vi "IsAnyOfType.vi"(8 "error in (no error)":errorcluster, 9 "Message Type":string, 10 "Any":T1, 11 "gRPCid in":T2) -> (0 "error out":errorcluster, 1 "Is Type":bool, 3 "gRPCid":T2)   [LabVIEW 2019, in "TestDataMarshal.lvlib" / "gprc-lvsupport.lvlib"]
uses:
  gprc-lvsupport.lvlib
  typeDefs/grpcId.ctl
  typeDefs/Any.ctl
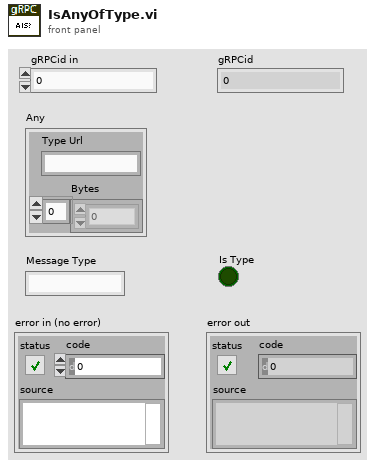
[diagram p1: front panel]
types:
  T1 = typedef "TestDataMarshal.lvlib/gprc-lvsupport.lvlib/Any.ctl" = cluster{"Type Url":string, "Bytes":u8[]}
  T2 = typedef "TestDataMarshal.lvlib/gprc-lvsupport.lvlib/grpcId.ctl" = u64
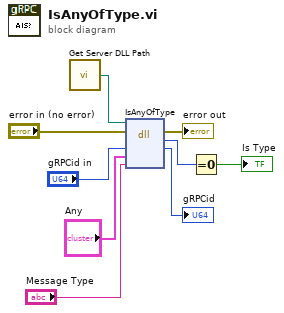
[diagram p0: block diagram]
diagram:
  n1 = call "Get Server DLL Path.vi"() -> ("Server dll path"=w8:path)
  n2 = dll-call lib="?" fn="IsAnyOfType"(path in=w8, error in="error in (no error)", "gRPCId"="gRPCid in", "any"="Any", "messageType"="Message Type") -> (error out=→"error out":errorcluster, "return type"=w3:i32, "gRPCId"=→"gRPCid":u64)  [unwired: 3 in, 1 out]
  n3 = Equal To 0?(x=w3) -> (x = 0?=→"Is Type":bool)
